vi "From Modbus To Veristand.vi"(7 "Parameters":T1={"Interface Data"={"Name"="", "Unit ID"=0, "Refresh Rate"=0, "Write Rate"=0, "Write Mode"=enum."Value Change", "Interface Type"=enum."TCP Master", "TCP Settings"={"Address"="", "Port"=0, "Timeout"=0}, "Serial Settings"={"VISA resource name"="", "baud rate"=0, "parity (even)"=0, "flow control (none)"=0, "serial type"=enum."RTU", "Wire Mode"=-1}}, "Modbus Input Groups"=[], "Modbus Output Groups"=[], "error in (no error)"={"status"=FALSE, "code"=0, "source"=""}, "Modbus Input Engine Group Names"=[], "Modbus Output Engine Group Names"=[]} {"Interface Data"."Serial Settings"."Wire Mode" items=["Unknown"=-1, "RS485/Wire4"=0, "RS485/Wire2-EchoDTR"=1, "RS485/Wire2-CtrlDTR"=2, "RS485/Wire2-Auto"=3, "RS232/DTE"=128, "RS232/DCE"=129, "RS232/AUTO"=130]; "Interface Data"."Serial Settings"."parity (even)" items=["None", "Odd", "Even", "Mark", "Space"]; "Interface Data"."Serial Settings"."flow control (none)" items=["None", "XON/XOFF", "RTS/CTS", "XON/XOFF & RTS/CTS", "DTR/DSR", "XON/XOFF & DTR/DSR"]}, 8 "error in (no error)":errorcluster, 10 "Process in":refnum<class "Process.lvclass">, 11 "Modbus API.lvlibp:Modbus Master":refnum<class "Modbus Master.lvclass">=refnum) -> ()   [LabVIEW 2020, in "Modbus Master Engine.lvlib"]
uses:
  Modbus Master Engine.lvlib
  <vilib>/NI/NIVS Inline Async API/_VS Inline Async API/Process/Process.lvclass
  <vilib>/NI/NIVS Inline Async API/_Data Access Engine/Data Access Engine/Data Access Engine.lvclass
  <vilib>/NI/NIVS Inline Async API/_Data Access Engine/Data Access Engine/Methods/Write.Data.vi
  <vilib>/NI/NIVS Inline Async API/_Data Access Engine/Data Access Engine/Methods/Write.Lookup.vi
  <vilib>/NI/NIVS Inline Async API/_Data Access Engine/Access Type Classes/Write/Write.lvclass
  Shared/Controls/Interface Type.ctl
  Shared/Modbus Master Shared.lvlib
  Shared/Controls/Data Model/TCP Settings.ctl
  Shared/Controls/Data Model/Serial Settings.ctl
  System Explorer/SubVIs/Modbus Type.ctl
  Shared/Controls/Data Model/DataType.ctl
  <vilib>/NI VeriStand/Custom Device API/Custom Device Item Ref.ctl
  <vilib>/NI VeriStand/Custom Device API/Custom Device API.lvlib
  Shared/Controls/Data Model/Mapping.ctl
  <vilib>/NI VeriStand/Custom Device API/Custom Device Channel Type.ctl
  Shared/Controls/Data Model/Channel.ctl
  Bulk Data Access.ctl
  Shared/Device Info.ctl
  Modbus API.lvlibp/API/Master/Modbus Master.lvclass
  Shared/Write Mode.ctl
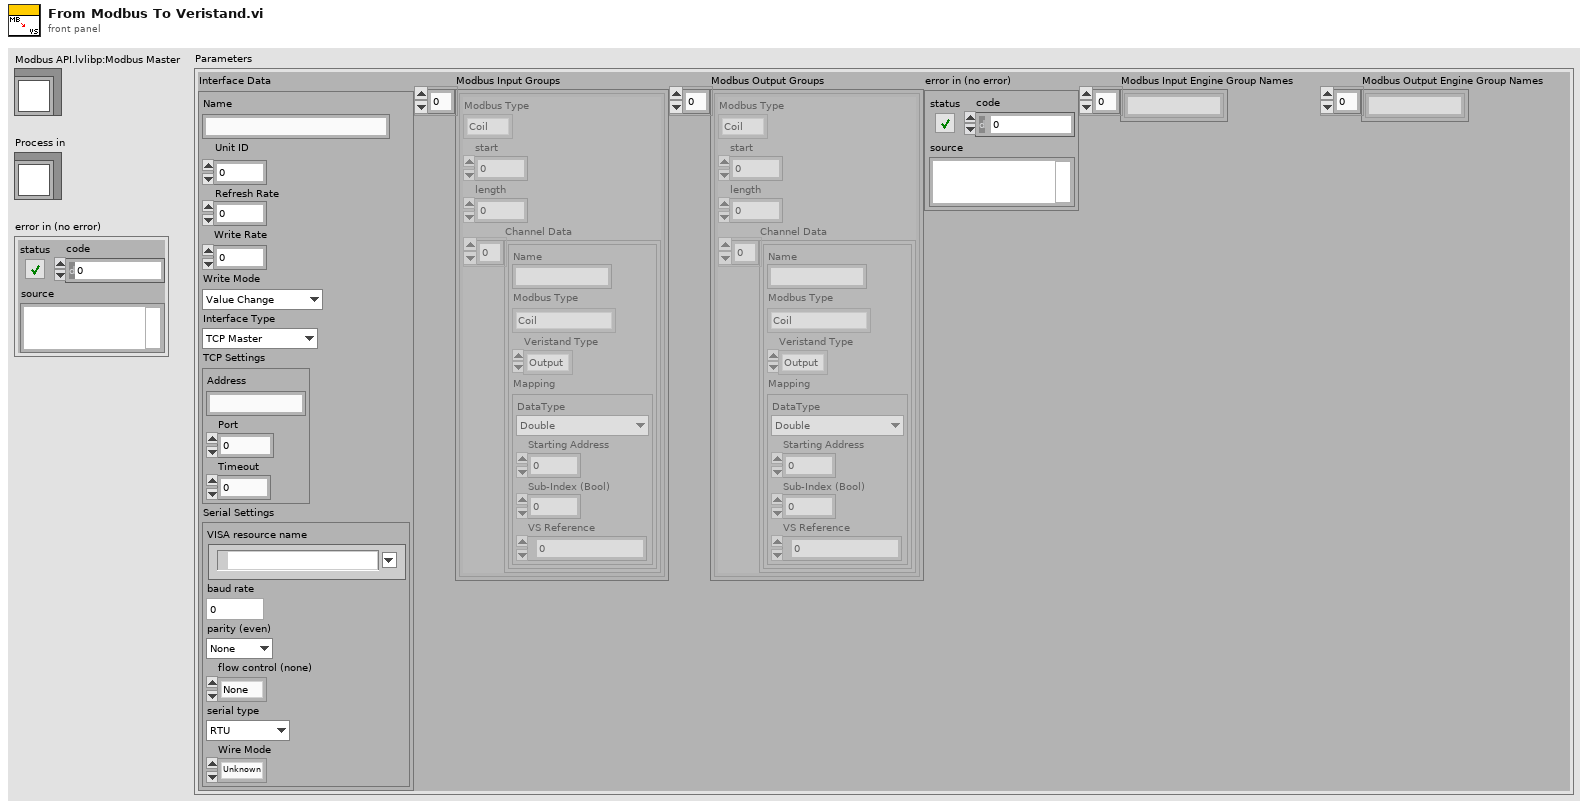
[diagram p1: front panel]
types:
  T1 = typedef "Modbus Master Shared.lvlib/Device Info.ctl" = cluster{"Interface Data":cluster{"Name":string, "Unit ID":u8, "Refresh Rate":i32, "Write Rate":i32, "Write Mode":T2, "Interface Type":T3, "TCP Settings":T4, "Serial Settings":T5}, "Modbus Input Groups":T6[], "Modbus Output Groups":T6[], "error in (no error)":errorcluster, "Modbus Input Engine Group Names":string[], "Modbus Output Engine Group Names":string[]}
  T2 = typedef "Modbus Master Shared.lvlib/Write Mode.ctl" = enum16{"Value Change", "Interval"}
  T3 = typedef "Modbus Master Shared.lvlib/Interface Type.ctl" = enum16{"TCP Master", "Serial Master", "TCP Slave", "Serial Slave"}
  T4 = typedef "Modbus Master Shared.lvlib/TCP Settings.ctl" = cluster{"Address":string, "Port":u16, "Timeout":i32}
  T5 = typedef "Modbus Master Shared.lvlib/Serial Settings.ctl" = cluster{"VISA resource name":refnum<visa-resource-name>, "baud rate":u32, "parity (even)":u16, "flow control (none)":u16, "serial type":enum16{"RTU", "ASCII"}, "Wire Mode":i16}
  T6 = typedef "Modbus Master Shared.lvlib/Bulk Data Access.ctl" = cluster{"Modbus Type":T7, "start":u16, "length":u16, "Channel Data":T8[]}
  T7 = typedef "Modbus Master Shared.lvlib/Modbus Type.ctl" = enum16{"Coil", "Discrete Input", "Holding Register", "Input Register"}
  T8 = typedef "Modbus Master Shared.lvlib/Channel.ctl" = cluster{"Name":string, "Modbus Type":T7, "Veristand Type":T9, "Mapping":T10}
  T9 = typedef "Custom Device API.lvlib/Custom Device Channel Type.ctl" = enum16{"Input", "Output"}
  T10 = typedef "Modbus Master Shared.lvlib/Mapping.ctl" = cluster{"DataType":T11, "Starting Address":u16, "Sub-Index (Bool)":u16, "VS Reference":T12}
  T11 = typedef "Modbus Master Shared.lvlib/DataType.ctl" = enum16{"Double", "Single", "I64", "I32", "I16", "I8", "U64", "U32", "U16", "U8", "Boolean"}
  T12 = typedef "Custom Device API.lvlib/Custom Device Item Ref.ctl" = u64
  T13 = typedef "Data Access Engine.lvlib/Data Access Engine.lvclass/Write.DVR.ctl" = refnum<data-value>
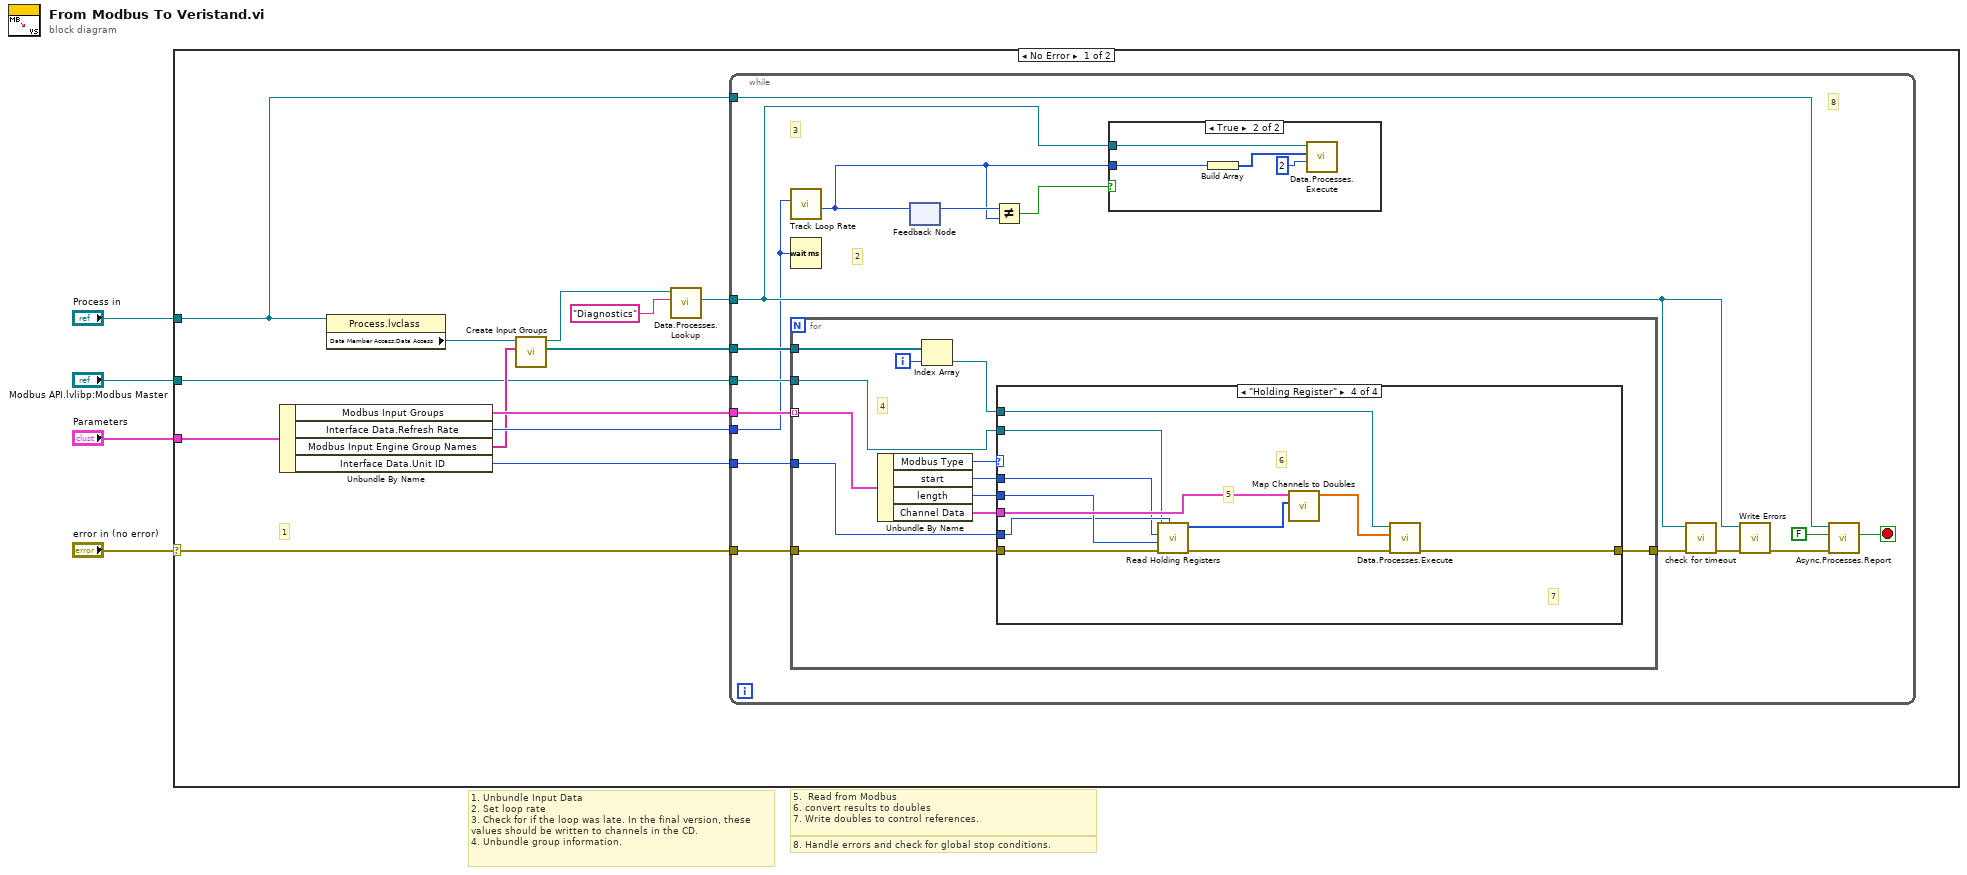
[diagram p0: block diagram]
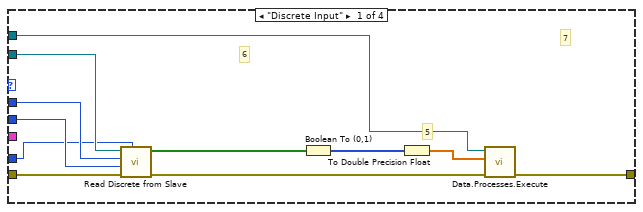
[diagram p3: hidden frame]
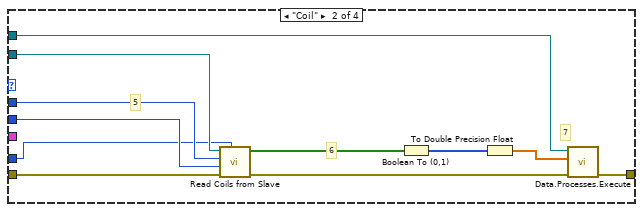
[diagram p4: hidden frame]
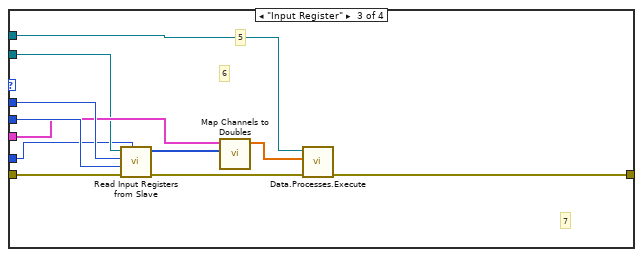
[diagram p5: hidden frame]
diagram:
  # "1. Unbundle Input Data\n2. Set loop rate\n3. Check for if the loop was late. In the final version, these\nvalues should be written to channels in the CD.\n4. Unbundle group information."
  # "5.  Read from Modbus\n6. convert results to doubles\n7. Write doubles to control references."
  # "8. Handle errors and check for global stop conditions."
  n1 = case shown="No Error" "error in (no error)" {
    selector: "error in (no error)" -> [w14 _]
    tunnel: "Parameters" -> [w15 _]
    tunnel: "Process in" -> [w13 _]
    tunnel: "Modbus API.lvlibp:Modbus Master" -> [w6 _]
    frame No Error {
      # "1"
      n2 = Unbundle By Name(w15) -> ("Modbus Input Groups"=w16:T6[], "Interface Data.Refresh Rate"=w17:i32, "Modbus Input Engine Group Names"=w11:string[], "Interface Data.Unit ID"=w5:u8)
      n3 = property class="Process.lvclass"(reference=w13) -> ("Data Member Access:Data Access"=w12:refnum<class "Data Access Engine.lvclass">)  [unwired: 1 in, 2 out]
      n4 = call "Create Input Groups.vi"("Output Engine Group Names"=w11, "Data Access Engine in"=w12) -> ("Array"=w10:T13[], "Data Access Engine out"=w8:refnum<class "Data Access Engine.lvclass">)  [unwired: 7 in, 1 out]
      n5 = call-poly <vilib>:"Data.Processes.Lookup.vi"("Name"="Diagnostics", "Data Access API in"=w8) -> ("Ref"=w7:T13)  [unwired: 6 in, 3 out]
      n6 = while {
        tunnel: w14 -> [w21]
        tunnel: w13 -> [w33]
        tunnel: w6 -> [w20]
        tunnel: w16 -> [w32]
        tunnel: w10 -> [w31]
        tunnel: w17 -> [w18]
        tunnel: w7 -> [w24]
        tunnel: w5 -> [w19]
        stop <- w30 stop-if-true
        # "8"
        # "3"
        # "2"
        n7 = call "Track Loop Rate.vi"("Refresh Rate"=w18) -> ("Late Count"=w26:i32)  [unwired: 8 in, 2 out]
        n8 = Wait (ms)(milliseconds to wait=w18) -> ()  [unwired: 1 out]
        n9 = for {
          tunnel: w32 -> [w49] mode=indexing
          tunnel: w31 -> [w44]
          tunnel: w20 -> [w47]
          tunnel: w21 -> [w39]
          tunnel: [w40] -> w23
          tunnel: w19 -> [w38]
          i -> [w42]
          # "4"
          n10 = Unbundle By Name(w49) -> ("Modbus Type"=w48:T7, "start"=w46:u16, "length"=w45:u16, "Channel Data"=w41:T8[])
          n11 = Index Array(array=w44, index=w42) -> (element=w43:T13)
          n12 = case shown="\"Holding Register\"" w48 {
            tunnel: w47 -> [w52 w63 w74 w84]
            tunnel: w46 -> [w56 w65 w81 w83]
            tunnel: w45 -> [w60 w64 w80 w88]
            tunnel: w39 -> [w51 w62 w73 w86]
            tunnel: [w58 w71 w82 w93] -> w40
            tunnel: w43 -> [w55 w70 w79 w92]
            tunnel: w41 -> [_ _ w77 w91]
            tunnel: w38 -> [w50 w61 w72 w85]
            frame "Discrete Input" {
              # "7"
              # "6"
              # "5"
              n13 = call "Read Discrete from Slave.vi"("Unit ID"=w50, "error in (no error)"=w51, "length"=w60, "start"=w56, "Modbus Master in"=w52) -> ("error out"=w59:errorcluster, "discrete inputs"=w57:bool[])  [unwired: 5 in]
              n14 = Boolean To (0,1)(Boolean=w57) -> (0, 1=w53:i16[])
              n15 = To Double Precision Float(number=w53) -> (double precision float=w54:dbl[])
              n16 = call-poly <vilib>:"Data.Processes.Execute.vi"("error in (no error)"=w59, "Values"=w54, "Ref"=w55) -> ("error out"=w58:errorcluster)  [unwired: 8 in]
            }
            frame "Coil" {
              # "7"
              # "6"
              # "5"
              n17 = call "Read Coils from Slave.vi"("Unit ID"=w61, "error in (no error)"=w62, "length"=w64, "start"=w65, "Modbus Master in"=w63) -> ("error out"=w67:errorcluster, "coils"=w66:bool[])  [unwired: 5 in]
              n18 = Boolean To (0,1)(Boolean=w66) -> (0, 1=w68:i16[])
              n19 = To Double Precision Float(number=w68) -> (double precision float=w69:dbl[])
              n20 = call-poly <vilib>:"Data.Processes.Execute.vi"("error in (no error)"=w67, "Values"=w69, "Ref"=w70) -> ("error out"=w71:errorcluster)  [unwired: 8 in]
            }
            frame "Input Register" {
              # "7"
              # "6"
              # "5"
              n21 = call "Read Input Registers from Slave.vi"("Unit ID"=w72, "error in (no error)"=w73, "length"=w80, "start"=w81, "Modbus Master in"=w74) -> ("error out"=w78:errorcluster, "register values"=w76:u16[])  [unwired: 5 in]
              n22 = call "Map Channels to Doubles.vi"("register values"=w76, "Channel Data"=w77) -> ("Array"=w75:dbl[])  [unwired: 9 in]
              n23 = call-poly <vilib>:"Data.Processes.Execute.vi"("error in (no error)"=w78, "Values"=w75, "Ref"=w79) -> ("error out"=w82:errorcluster)  [unwired: 8 in]
            }
            frame "Holding Register" {
              # "7"
              # "6"
              # "5"
              n24 = call "Read Holding Registers.vi"("Unit ID"=w85, "error in (no error)"=w86, "length"=w88, "start"=w83, "Modbus Master in"=w84) -> ("error out"=w87:errorcluster, "register values"=w89:u16[])  [unwired: 5 in]
              n25 = call "Map Channels to Doubles.vi"("register values"=w89, "Channel Data"=w91) -> ("Array"=w90:dbl[])  [unwired: 9 in]
              n26 = call-poly <vilib>:"Data.Processes.Execute.vi"("error in (no error)"=w87, "Values"=w90, "Ref"=w92) -> ("error out"=w93:errorcluster)  [unwired: 8 in]
            }
          }
        }
        n27 = feedback-in #1(w26) -> ()
        n28 = feedback #1() -> (w28:i32)  [unwired: 1 in]
        n29 = Not Equal?(x=w28, y=w26) -> (x != y?=w27:bool)
        n30 = case shown="True" w27 {
          tunnel: w24 -> [_ w37]
          tunnel: w26 -> [_ w35]
          frame False {
          }
          frame True {
            n31 = Build Array(w35) -> (w34:i32[])
            n32 = call-poly <vilib>:"Data.Processes.Execute.vi"("Offset"=2, "Values"=w34, "Ref"=w37) -> ()  [unwired: 8 in, 1 out]
          }
        }
        n33 = call "check for timeout.vi"("error in (no error)"=w23, "Data Value Reference in"=w24) -> ("error out"=w22:errorcluster)  [unwired: 9 in]
        n34 = call "Write Errors.vi"("error in (no error)"=w22, "Data Value Reference in"=w24) -> ("error out"=w25:errorcluster)  [unwired: 9 in]
        n35 = call <vilib>:"Async.Processes.Report.vi"("Error"=w25, "Stop Async on Error?"=FALSE ("Stop on Error?"), "Process in"=w33) -> ("Stop"=w30:bool)  [unwired: 7 in, 1 out]
      }
    }
    frame Error {
    }
  }
